vi "_vna_simpleSweep_(R&S_sweepMagPhase_sub).vi"(0 "Boolean":bool=TRUE, 1 "Sweep Type":i32(ring) caption="Sweep Type:" items=["Lin. Frequency", "Log. Frequency", "Segmented Frequency", "Power", "CW Mode", "Time"], 2 "Points:":i32=201, 5 "Power dBm":dbl=-25.0 caption="Power, dBm" format="%#.3f", 7 "Center Freq:":dbl=3090000000.0 format="%^#.6e", 9 "Span Freq:":dbl=400000000.0 format="%^#.3e", 11 "Bandwidth:":dbl=1.0 caption="Bandwidth (1 to 1e6 Hz):" format="%#.3f", 12 "Fast sweep?":bool) -> (6 "Lin Mag":cluster{dbl[], dbl[]}(graph), 8 "Phase":cluster{dbl[], dbl[]}(graph))   [LabVIEW 2013]
uses:
  <instrlib>/Rohde&Schwarz Vector Network Analyzer/Rohde&Schwarz Vector Network Analyzer.lvlib
panel:
  out "Trace Name":string="Trc1"
  out "Channel Number":i32=1
  in  "Trace":i32=1
  in  "Out Port:":i32=2
  in  "In Port:":i32=1
  in  "Sweep Mode Continuous (Off)":bool
  out "No of Values Stimulus":i32=201
  out "No of Values Responce":i32=402
  out "curve number":i32=1
  in  "Stop":bool
  # "R&S VNA"
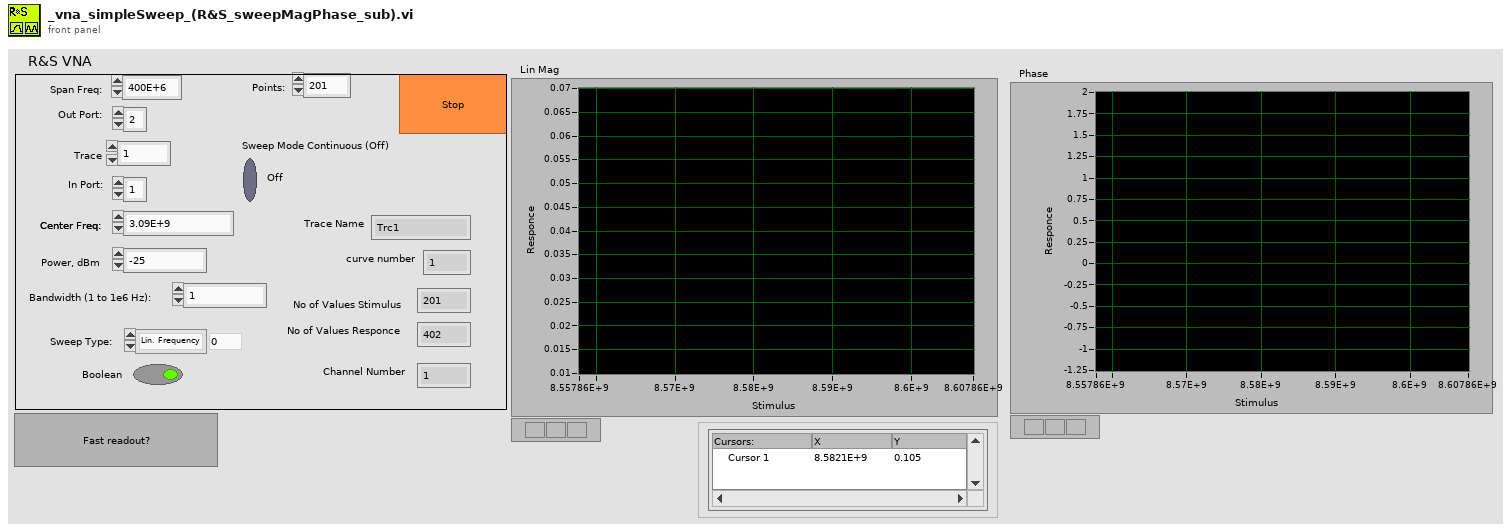
[diagram p1: front panel]
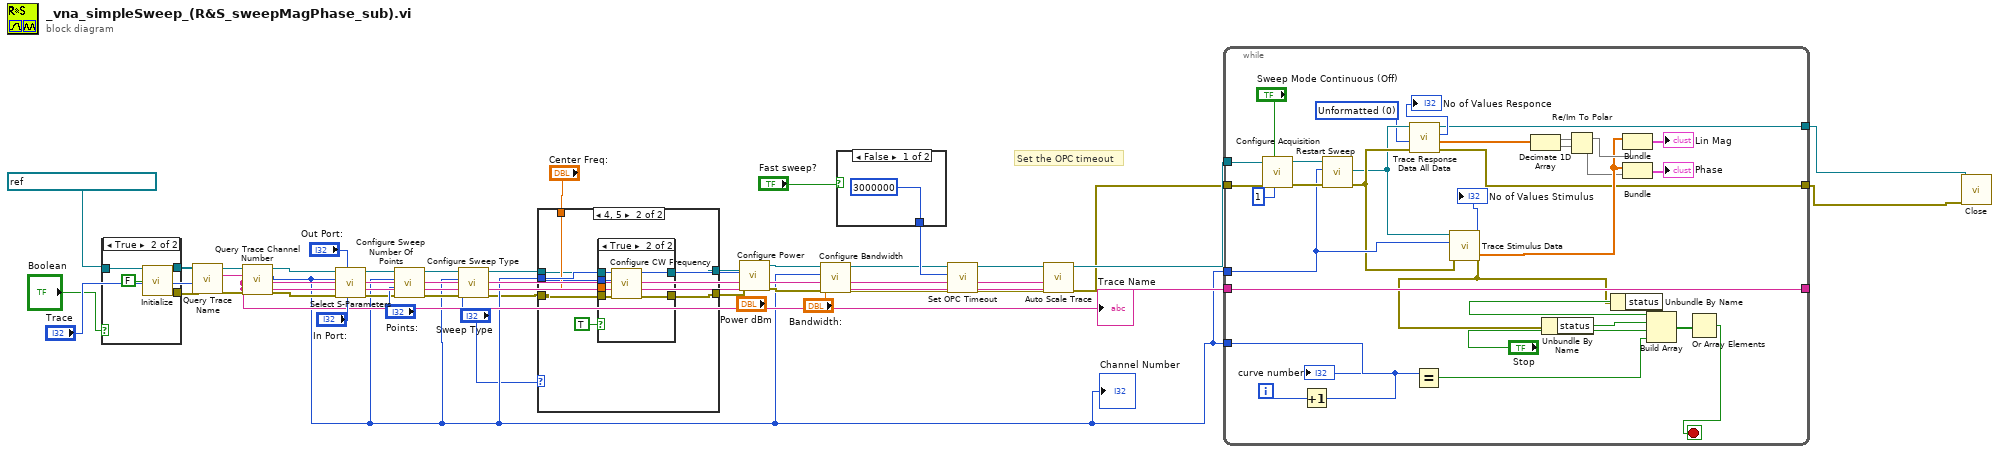
[diagram p0: block diagram]
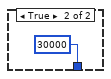
[diagram p2: hidden frame]
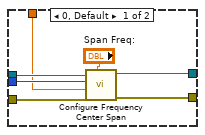
[diagram p3: hidden frame]
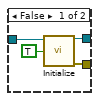
[diagram p5: hidden frame]
diagram:
  # "Set the OPC timeout"
  n1 = case shown="True" "Boolean" {
    tunnel: [w39 w46] -> w32
    tunnel: [w40 w45] -> w31
    tunnel: refnum<visa-resource-name> "TCPIP::192.168.0.3::INST" ("VISA resource name") -> [w41 w44]
    frame False {
      n2 = call <instrlib>:"Initialize.vi"("VISA resource name"=w41, "Reset (T: Reset)"=TRUE) -> ("VISA resource name out"=w40:refnum<visa-resource-name>, "error out"=w39:errorcluster)  [unwired: 12 in]
    }
    frame True {
      n3 = call <instrlib>:"Initialize.vi"("VISA resource name"=w44, "Reset (T: Reset)"=FALSE) -> ("VISA resource name out"=w45:refnum<visa-resource-name>, "error out"=w46:errorcluster)  [unwired: 12 in]
    }
  }
  n4 = call <instrlib>:"Query Trace Name.vi"("error in (no error)"=w32, "Trace Number (1)"="Trace", "VISA resource name"=w31) -> ("error out"=w34:errorcluster, "Trace Name"=w18:string, "VISA resource name out"=w33:refnum<visa-resource-name>)  [unwired: 6 in]
  "Trace Name" <- w18
  n5 = call <instrlib>:"Query Trace Channel Number.vi"("error in (no error)"=w34, "Trace Name (\"Ch2Trc2\")"=w18, "VISA resource name"=w33) -> ("error out"=w36:errorcluster, "Channel Number"=w11:i32, "VISA resource name out"=w35:refnum<visa-resource-name>)  [unwired: 6 in]
  "Channel Number" <- w11
  n6 = call <instrlib>:"Select S-Parameters.vi"("In Port (1)"="In Port:", "Out Port (1)"="Out Port:", "error in (no error)"=w36, "Channel (1)"=w11, "VISA resource name"=w35) -> ("error out"=w12:errorcluster, "VISA resource name out"=w13:refnum<visa-resource-name>)  [unwired: 5 in]
  n7 = call <instrlib>:"Configure Sweep Number Of Points.vi"("error in (no error)"=w12, "Number Of Points (201)"="Points:", "Channel (1)"=w11, "VISA resource name"=w13) -> ("error out"=w15:errorcluster, "VISA resource name out"=w16:refnum<visa-resource-name>)  [unwired: 6 in]
  n8 = call <instrlib>:"Configure Sweep Type.vi"("error in (no error)"=w15, "Sweep Type (Power)"="Sweep Type", "Channel (1)"=w11, "VISA resource name"=w16) -> ("error out"=w8:errorcluster, "VISA resource name out"=w9:refnum<visa-resource-name>)  [unwired: 6 in]
  n9 = case shown="4, 5" "Sweep Type" {
    tunnel: [w53 w58] -> w29
    tunnel: [w52 w56] -> w28
    tunnel: w9 -> [w50 w59]
    tunnel: w8 -> [w49 w57]
    tunnel: w11 -> [w48 w55]
    tunnel: "Center Freq:" -> [w47 w60]
    frame 0, Default {
      n10 = call <instrlib>:"Configure Frequency Center Span.vi"("Span (300.0e3)"="Span Freq:", "error in (no error)"=w49, "Center Frequency (4.0e9)"=w47, "Channel (1)"=w48, "VISA resource name"=w50) -> ("error out"=w52:errorcluster, "VISA resource name out"=w53:refnum<visa-resource-name>)  [unwired: 5 in]
    }
    frame 4, 5 {
      n11 = case shown="True" TRUE {
        tunnel: w60 -> [_ w68]
        tunnel: w59 -> [w62 w67]
        tunnel: [w62 w66] -> w58
        tunnel: w57 -> [w61 w65]
        tunnel: [w61 w64] -> w56
        tunnel: w55 -> [_ w63]
        frame False {
        }
        frame True {
          n12 = call <instrlib>:"Configure CW Frequency.vi"("error in (no error)"=w65, "CW Frequency (1.0e9)"=w68, "Channel (1)"=w63, "VISA resource name"=w67) -> ("error out"=w64:errorcluster, "VISA resource name out"=w66:refnum<visa-resource-name>)  [unwired: 6 in]
        }
      }
    }
  }
  n13 = call <instrlib>:"Configure Power.vi"("error in (no error)"=w28, "Power (-10.0)"="Power dBm", "Channel (1)"=w11, "VISA resource name"=w29) -> ("error out"=w26:errorcluster, "VISA resource name out"=w27:refnum<visa-resource-name>)  [unwired: 6 in]
  n14 = call <instrlib>:"Configure Bandwidth.vi"("error in (no error)"=w26, "Bandwidth (10.0e3)"="Bandwidth:", "Channel (1)"=w11, "VISA resource name"=w27) -> ("error out"=w4:errorcluster, "VISA resource name out"=w5:refnum<visa-resource-name>)  [unwired: 6 in]
  n15 = case shown="False" "Fast sweep?" {
    tunnel: [3000000 ("OPC Timeout (30000)") 30000 ("OPC Timeout (30000)")] -> w6
    frame False {
    }
    frame True {
    }
  }
  n16 = call <instrlib>:"Set OPC Timeout.vi"("error in (no error)"=w4, "OPC Timeout"=w6, "VISA resource name"=w5) -> ("error out"=w3:errorcluster, "VISA resource name out"=w2:refnum<visa-resource-name>)  [unwired: 7 in]
  n17 = call <instrlib>:"Auto Scale Trace.vi"("error in (no error)"=w3, "Trace Name (\"\")"=w18, "VISA resource name"=w2) -> ("error out"=w19:errorcluster, "VISA resource name out"=w20:refnum<visa-resource-name>)  [unwired: 7 in]
  n18 = while {
    tunnel: w20 -> [w94]
    tunnel: w19 -> [w93]
    tunnel: w11 -> [w88]
    tunnel: w11 -> [w103]
    tunnel: w18 -> [w96]
    tunnel: [w96] -> _
    tunnel: [w75] -> w38
    tunnel: [w74] -> w37
    i -> [w95]
    stop <- w71 stop-if-true
    w85 = 0 items=["Unformatted", "Formatted", "Unformatted With Trace Mathematics"] ("Data Format (Unformatted)")
    n19 = call <instrlib>:"Configure Acquisition.vi"("Sweep Count (1)"=1, "Sweep Mode Continuous (Off)"="Sweep Mode Continuous (Off)", "error in (no error)"=w93, "VISA resource name"=w94) -> ("error out"=w90:errorcluster, "VISA resource name out"=w91:refnum<visa-resource-name>)  [unwired: 6 in]
    n20 = Increment(x=w95) -> (x+1=w72:i32)
    "curve number" <- w72
    n21 = call <instrlib>:"Restart Sweep.vi"("error in (no error)"=w90, "Channel (1)"=w88, "VISA resource name"=w91) -> ("error out"=w87:errorcluster, "VISA resource name out"=w86:refnum<visa-resource-name>)  [unwired: 7 in]
    n22 = call <instrlib>:"Trace Response Data All Data.vi"("error in (no error)"=w87, "Data Format (Unformatted)"=w85, "VISA resource name"=w86) -> ("error out"=w74:errorcluster, "Trace Data"=w84:dbl[], "No of Values"=→"No of Values Responce":i32, "VISA resource name out"=w75:refnum<visa-resource-name>)  [unwired: 5 in]
    n23 = Equal?(x=w103, y=w72) -> (x = y?=w99:bool)
    n24 = call <instrlib>:"Trace Stimulus Data.vi"("error in (no error)"=w87, "Channel (1)"=w88, "VISA resource name"=w86) -> ("error out"=w73:errorcluster, "Trace Data"=w79:dbl[], "No of Values"=→"No of Values Stimulus":i32)  [unwired: 5 in, 1 out]
    n25 = Decimate 1D Array(w84) -> (w82:dbl[], w81:dbl[])
    n26 = Unbundle By Name(w73) -> ("status"=w101:bool)
    n27 = Re/Im To Polar(2:w81, 3:w82) -> (0:w78:dbl[], 1:w80:dbl[])
    n28 = Unbundle By Name(w73) -> ("status"=w102:bool)
    n29 = Bundle("Trace Data"=w79, w80) -> (→"Lin Mag":cluster{"Trace Data":dbl[], dbl[]})  [unwired: 1 in]
    n30 = Bundle("Trace Data"=w79, w78) -> (→"Phase":cluster{"Trace Data":dbl[], dbl[]})  [unwired: 1 in]
    n31 = Build Array(w102, w101, "Stop", w99) -> (w98:bool[])
    n32 = Or Array Elements(Boolean array=w98) -> (logical OR=w71:bool)
  }
  n33 = call <instrlib>:"Close.vi"("error in (no error)"=w37, "VISA resource name"=w38) -> ()  [unwired: 9 in, 1 out]
